vi "Write Drag Timeout.vi"(8 "error in (no error)":errorcluster, 10 "Drag Timeout":i32, 11 "QMenu Class in":refnum<class "QMenu Class.lvclass">) -> (0 "error out":errorcluster, 3 "QMenu Class out":refnum<class "QMenu Class.lvclass">)   [LabVIEW 2020, in "QTab.lvlib" / "QMenu Class.lvclass"]
uses:
  QMenu Class.lvclass
  QMenu Class.lvclass/QMenu Class.ctl
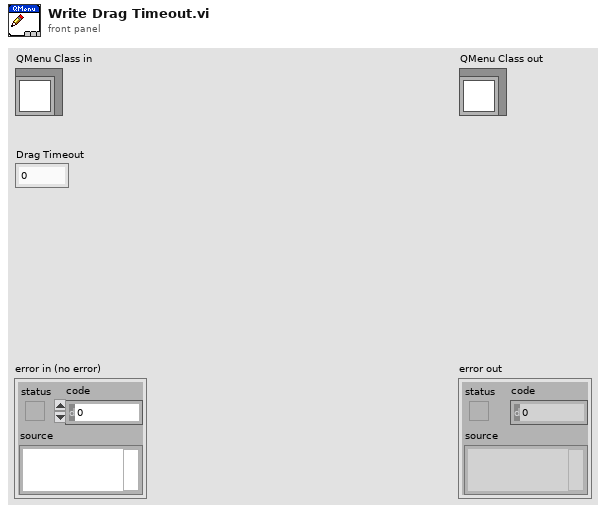
[diagram p1: front panel]
types:
  T1 = typedef "QTab.lvlib/QMenu Class.lvclass/Parameter.ctl" = cluster{"Close Timeout":i32, "Drag Timeout":i32}
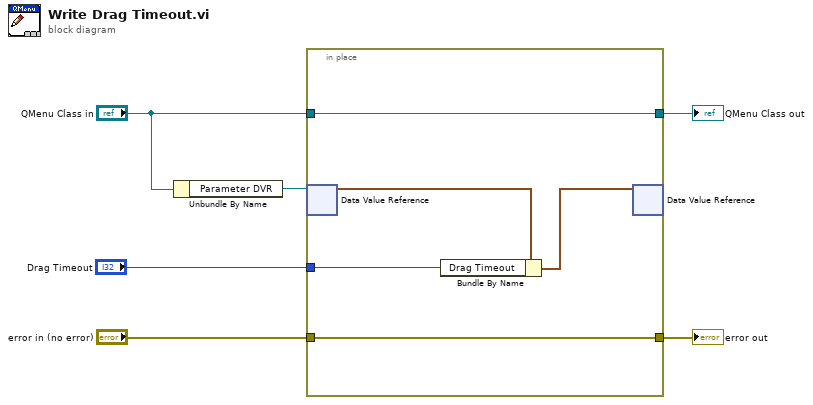
[diagram p0: block diagram]
diagram:
  n1 = Unbundle By Name("QMenu Class in") -> ("Parameter DVR"=w6:refnum<data-value>)
  n2 = in-place {
    in-place-border: "QMenu Class in" -> [w11]
    in-place-border: "error in (no error)" -> [w10]
    in-place-border: [w11] -> w3
    in-place-border: [w10] -> w2
    in-place-border: "Drag Timeout" -> [w8]
    n3 = in-place-dvr #1(w6) -> (w9:T1)  [unwired: 1 out]
    n4 = Bundle By Name(cluster=w9, "Drag Timeout"=w8) -> (w7:T1)
    n5 = in-place-dvr #1(w7) -> ()  [unwired: 2 out]
  }
  "error out" <- w2
  "QMenu Class out" <- w3
